vi "set_rectangle.vi"(0 "Set/Add":bool, 1 "Handle":i32, 2 "y2":dbl, 3 "x2":dbl, 4 "y1":dbl, 5 "x1":dbl) -> ()   [LabVIEW 2015]
uses:
  MWT.dll
panel:
  out "return type":i32
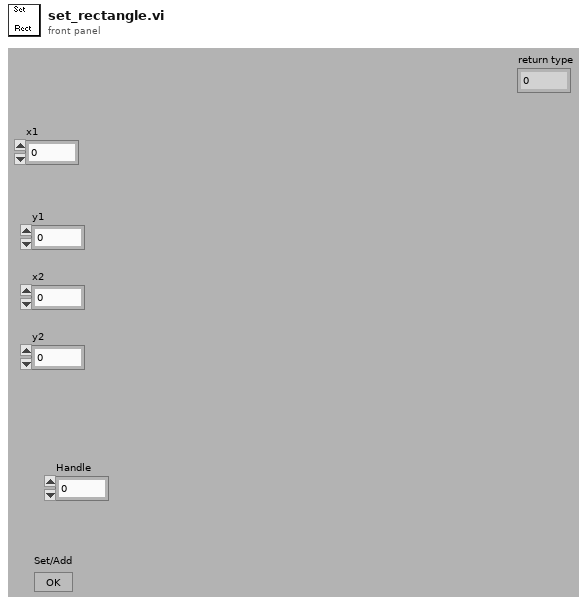
[diagram p1: front panel]
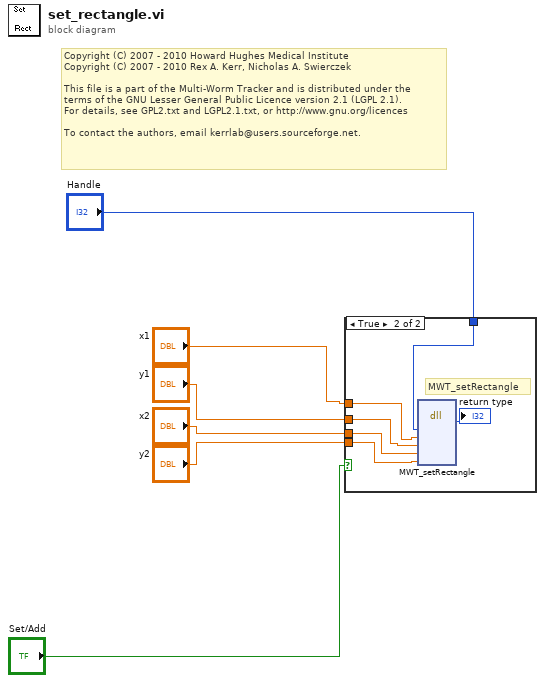
[diagram p0: block diagram]
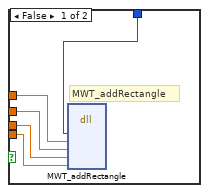
[diagram p2: hidden frame]
diagram:
  # "Copyright (C) 2007 - 2010 Howard Hughes Medical Institute\nCopyright (C) 2007 - 2010 Rex A. Kerr, Nicholas A. Swierczek\n \nThis file is a part of the Multi-Worm Tracker and is distributed under the\nterms of the GNU Lesser General Public Licence version 2.1 (LGPL 2.1).\nFor details, see GPL2.txt and LGPL2.1.txt, or http://www.gnu.org/licences\n \nTo contact the authors, email kerrlab@users.sourceforge.net."
  n1 = case shown="True" "Set/Add" {
    tunnel: "Handle" -> [w11 w17]
    tunnel: "y2" -> [w10 w13]
    tunnel: "x2" -> [w9 w14]
    tunnel: "y1" -> [w8 w15]
    tunnel: "x1" -> [w7 w16]
    frame False {
      # "MWT_addRectangle"
      n2 = dll-call lib="C:/Users/ramasamyl/Desktop/MWT/MWT.dll" fn="MWT_addRectangle"("handle"=w11, "x1"=w7, "y1"=w8, "x2"=w9, "y2"=w10) -> ()  [unwired: 9 in, 2 out]
    }
    frame True {
      # "MWT_setRectangle"
      n3 = dll-call lib="C:/Users/ramasamyl/Desktop/MWT/MWT.dll" fn="MWT_setRectangle"("handle"=w17, "left"=w16, "right"=w15, "top"=w14, "bottom"=w13) -> ("return type"=→"return type":i32)  [unwired: 8 in, 2 out]
    }
  }
